vi "Engine - Error - Initialization.vi"(8 "error in (no error)":errorcluster) -> (0 "error out":errorcluster, 2 "Runtime Status Channels Out":dbl[](array[numeric]))   [LabVIEW 2015, in "DMM-SWITCH-ScanList Engine.lvlib"]
uses:
  DMM-SWITCH-ScanList Engine.lvlib
panel:
  in  "Runtime Status Channels In":dbl[](array[numeric])
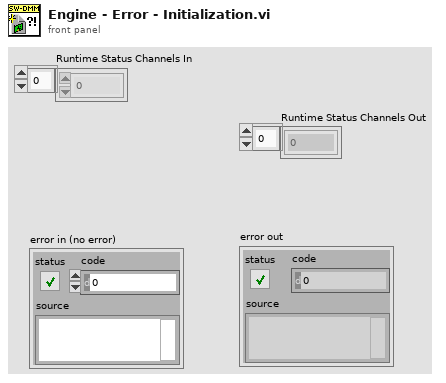
[diagram p1: front panel]
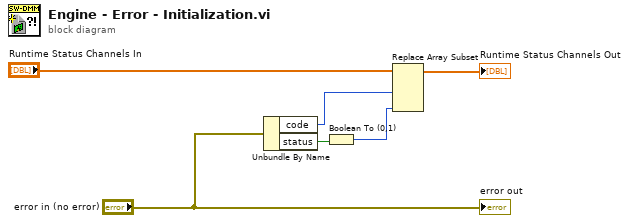
[diagram p0: block diagram]
diagram:
  n1 = Unbundle By Name("error in (no error)") -> ("code"=w3:i32, "status"=w5:bool)
  n2 = Boolean To (0,1)(Boolean=w5) -> (0, 1=w2:i16)
  n3 = Replace Array Subset(array="Runtime Status Channels In", new element #1=w3, new element #2=w2) -> (→"Runtime Status Channels Out":dbl[])  [unwired: 2 in]
  "error out" <- "error in (no error)"
